vi "Check Image Deplication.vi"(8 "error in (no error)":errorcluster, 11 "Actor in":refnum<class "Actor.lvclass">) -> (0 "error out":errorcluster, 3 "Actor out":refnum<class "Actor.lvclass">)   [LabVIEW 2015, in "Actor.lvclass"]
uses:
  Actor.lvclass
  Actor.lvclass/Actor.ctl
  FileOperation/FileOperation.lvclass
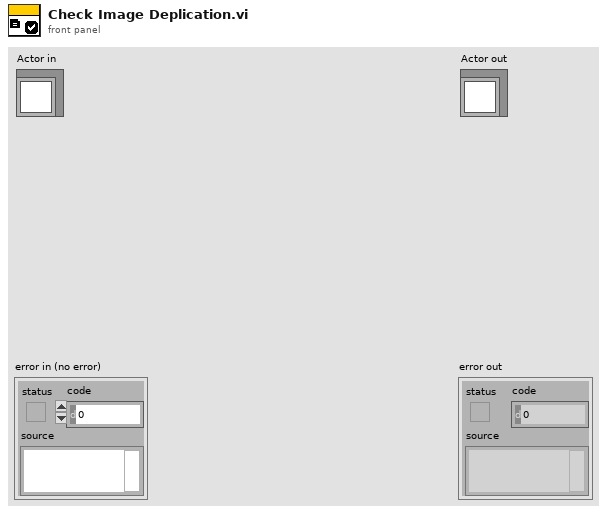
[diagram p1: front panel]
types:
  T1 = enum8{"Enabled", "Disabled", "Disabled and Grayed Out"}
  T2 = typedef "Actor.lvclass/Main Ctl and VI Refenerce.ctl" = cluster{"Size":refnum<vi>, "Save Path":refnum<vi>, "Slide":refnum<vi>, "Cut":refnum<vi>, "Previous Button":refnum<vi>, "Next Button":refnum<vi>, "This VI":refnum<vi>}
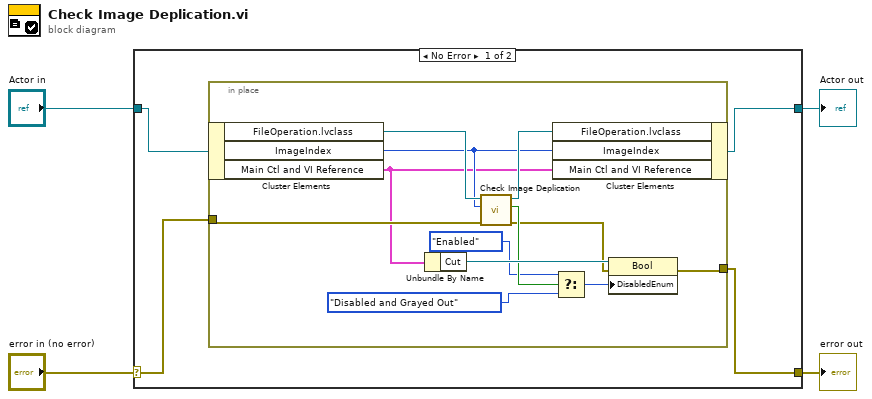
[diagram p0: block diagram]
diagram:
  n1 = case shown="No Error" "error in (no error)" {
    selector: "error in (no error)" -> [w7 w22]
    tunnel: [w5 w22] -> w3
    tunnel: [w6 w21] -> w1
    tunnel: "Actor in" -> [w8 w21]
    frame No Error {
      n2 = in-place {
        in-place-border: w7 -> [w18]
        in-place-border: [w10] -> w5
        n3 = in-place-cluster #1(w8) -> ("FileOperation.lvclass"=w20:refnum<class "FileOperation.lvclass">, "ImageIndex"=w17:i32, "Main Ctl and VI Reference"=w9:T2)
        n4 = Unbundle By Name(w9) -> ("Cut"=w16:refnum<vi>)
        n5 = call "Check Image Deplication.vi"("error in (no error)"=w18, "IndexOfImages"=w17, "FileOperation in"=w20) -> ("error out"=w11:errorcluster, "Effective?(True)"=w15:bool, "FileOperation out"=w19:refnum<class "FileOperation.lvclass">)  [unwired: 6 in]
        n6 = in-place-cluster #1("FileOperation.lvclass"=w19, "ImageIndex"=w17, "Main Ctl and VI Reference"=w9) -> (w6:refnum<class "Actor.lvclass">)
        n7 = Select(t=T1."Enabled" ("Disabled"), s=w15, f=T1."Disabled and Grayed Out" ("Disabled")) -> (s? t:f=w12:T1)
        n8 = property class="Bool"(reference=w16, error in=w11, "DisabledEnum"=w12) -> (error out=w10:errorcluster)  [unwired: 1 out]
      }
    }
    frame Error {
    }
  }
  "error out" <- w3
  "Actor out" <- w1
